vi "Create_Commands.vi"() -> ()   [LabVIEW 2012]
panel:
  out "error out":errorcluster
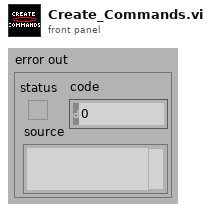
[diagram p1: front panel]
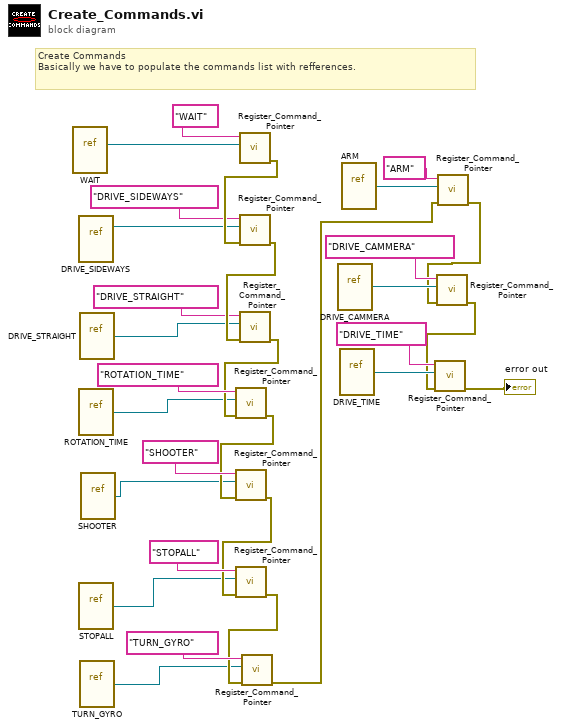
[diagram p0: block diagram]
diagram:
  # "Create Commands\nBasically we have to populate the commands list with refferences."
  n1 = vi-ref "WAIT.vi"() -> (w30:refnum<vi>)
  n2 = vi-ref "DRIVE_SIDEWAYS.vi"() -> (w24:refnum<vi>)
  n3 = vi-ref "ROTATION_TIME.vi"() -> (w16:refnum<vi>)
  n4 = vi-ref "STOPALL.vi"() -> (w14:refnum<vi>)
  n5 = vi-ref "DRIVE_STRAIGHT.vi"() -> (w23:refnum<vi>)
  n6 = vi-ref "TURN_GYRO.vi"() -> (w11:refnum<vi>)
  n7 = vi-ref "SHOOTER.vi"() -> (w15:refnum<vi>)
  n8 = call "Register_Command_Pointer.vi"("Strict-Typed VI Refnum"=w30, "Name"="WAIT" ("refnum name")) -> ("error out"=w28:errorcluster)  [unwired: 9 in]
  n9 = call "Register_Command_Pointer.vi"("error in (no error)"=w28, "Strict-Typed VI Refnum"=w24, "Name"="DRIVE_SIDEWAYS" ("refnum name")) -> ("error out"=w26:errorcluster)  [unwired: 8 in]
  n10 = call "Register_Command_Pointer.vi"("error in (no error)"=w26, "Strict-Typed VI Refnum"=w23, "Name"="DRIVE_STRAIGHT" ("refnum name")) -> ("error out"=w17:errorcluster)  [unwired: 8 in]
  n11 = call "Register_Command_Pointer.vi"("error in (no error)"=w17, "Strict-Typed VI Refnum"=w16, "Name"="ROTATION_TIME" ("refnum name")) -> ("error out"=w19:errorcluster)  [unwired: 8 in]
  n12 = call "Register_Command_Pointer.vi"("error in (no error)"=w19, "Strict-Typed VI Refnum"=w15, "Name"="SHOOTER" ("refnum name")) -> ("error out"=w21:errorcluster)  [unwired: 8 in]
  n13 = call "Register_Command_Pointer.vi"("error in (no error)"=w21, "Strict-Typed VI Refnum"=w14, "Name"="STOPALL" ("refnum name")) -> ("error out"=w12:errorcluster)  [unwired: 8 in]
  n14 = call "Register_Command_Pointer.vi"("error in (no error)"=w12, "Strict-Typed VI Refnum"=w11, "Name"="TURN_GYRO" ("refnum name")) -> ("error out"=w1:errorcluster)  [unwired: 8 in]
  n15 = vi-ref "DRIVE_CAMMERA.vi"() -> (w9:refnum<vi>)
  n16 = vi-ref "DRIVE_TIME.vi"() -> (w10:refnum<vi>)
  n17 = vi-ref "ARM.vi"() -> (w8:refnum<vi>)
  n18 = call "Register_Command_Pointer.vi"("error in (no error)"=w1, "Strict-Typed VI Refnum"=w8, "Name"="ARM") -> ("error out"=w2:errorcluster)  [unwired: 8 in]
  n19 = call "Register_Command_Pointer.vi"("error in (no error)"=w2, "Strict-Typed VI Refnum"=w9, "Name"="DRIVE_CAMMERA") -> ("error out"=w3:errorcluster)  [unwired: 8 in]
  n20 = call "Register_Command_Pointer.vi"("error in (no error)"=w3, "Strict-Typed VI Refnum"=w10, "Name"="DRIVE_TIME") -> ("error out"=→"error out":errorcluster)  [unwired: 8 in]
